vi "startContinuousMove.vi"(0 "connection ID in":refnum<k5>, 1 "axis":i32(ring) items=["1", "2", "3"], 2 "direction [t=bwd | f=fwd]":bool, 3 "start | stop":bool, 5 "error in":errorcluster) -> (14 "connection ID":refnum<k5>, 15 "axis_out":i32(ring) items=["1", "2", "3"], 19 "error out":errorcluster)   [LabVIEW 2016, in "AMC_VIs.lvlib"]
doc: "By means of this VI continuous movement on a specific axis either in forward or backward direction can be started or stopped."
uses:
  AMC_VIs.lvlib
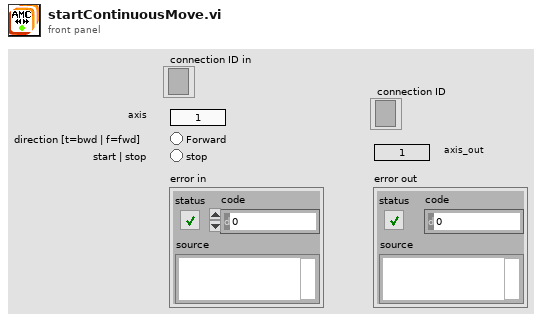
[diagram p1: front panel]
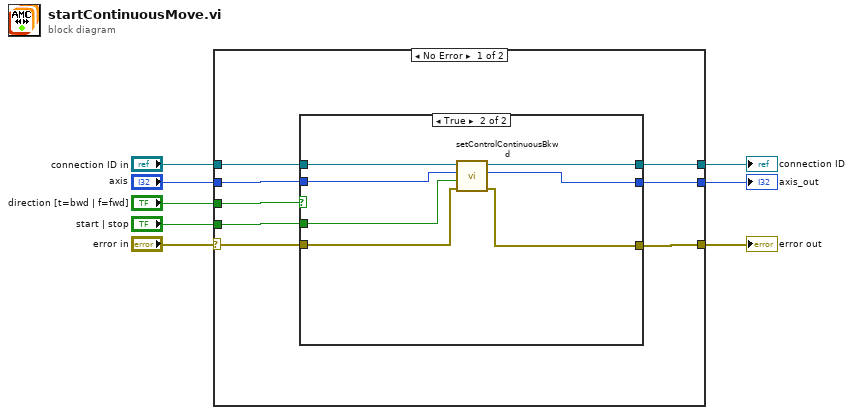
[diagram p0: block diagram]
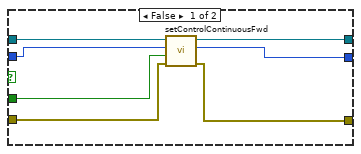
[diagram p2: hidden frame]
diagram:
  n1 = case shown="No Error" "error in" {
    selector: "error in" -> [w12 w31]
    tunnel: "connection ID in" -> [w16 w33]
    tunnel: "direction [t=bwd | f=fwd]" -> [w15 _]
    tunnel: "axis" -> [w14 w32]
    tunnel: "start | stop" -> [w13 _]
    tunnel: [w11 w31] -> w3
    tunnel: [w10 w32] -> w2
    tunnel: [w9 w33] -> w1
    frame No Error {
      n2 = case shown="True" w15 {
        tunnel: w16 -> [w23 w29]
        tunnel: w14 -> [w21 w30]
        tunnel: w13 -> [w20 w28]
        tunnel: w12 -> [w19 w27]
        tunnel: [w18 w26] -> w11
        tunnel: [w17 w25] -> w10
        tunnel: [w22 w24] -> w9
        frame False {
          n3 = call "setControlContinuousFwd.vi"("error in"=w19, "enable"=w20, "axis"=w21, "connection ID"=w23) -> ("error out"=w18:errorcluster, "axis_out"=w17:i32, "connection ID"=w22:refnum<k5>)  [unwired: 5 in]
        }
        frame True {
          n4 = call "setControlContinuousBkwd.vi"("error in"=w27, "enable"=w28, "axis"=w30, "connection ID"=w29) -> ("error out"=w26:errorcluster, "axis_out"=w25:i32, "connection ID"=w24:refnum<k5>)  [unwired: 5 in]
        }
      }
    }
    frame Error {
    }
  }
  "connection ID" <- w1
  "error out" <- w3
  "axis_out" <- w2
